vi "Points to [X] [Y].vi"(11 "Points":cluster{"X":dbl, "Y":dbl}[](array[cluster])) -> (2 "Y":dbl[](array[numeric]), 3 "X":dbl[](array[numeric]))   [LabVIEW 2020, in "AoC 2022.lvlib"]
uses:
  AoC 2022.lvlib
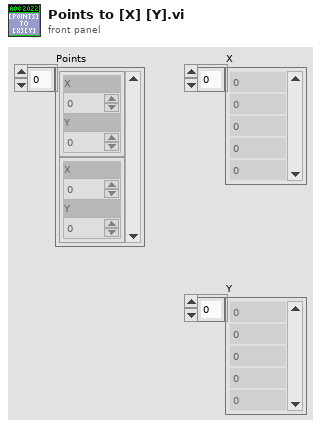
[diagram p1: front panel]
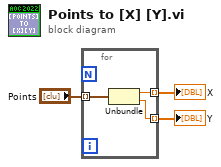
[diagram p0: block diagram]
diagram:
  n1 = for {
    tunnel: "Points" -> [w6] mode=indexing
    tunnel: [w5] -> w2 mode=indexing
    tunnel: [w4] -> w3 mode=indexing
    n2 = Unbundle(w6) -> ("X"=w5:dbl, "Y"=w4:dbl)
  }
  "Y" <- w3
  "X" <- w2
